vi "StartManageVIActivation.vi"(8 "error in (no error)":errorcluster, 11 "Menu in":refnum<class "VIActivation.lvclass">) -> (0 "error out":errorcluster, 3 "Menu out":refnum<class "VIActivation.lvclass">)   [LabVIEW 2021, in "VIActivation.lvlib" / "VIActivation.lvclass"]
uses:
  VIActivation.lvclass
  VIActivation.lvclass/VIActivation.ctl
  TR_ManageVIActivation.vi
  566083a2-3826-408d-bdf5-5786947dd1dc.vi
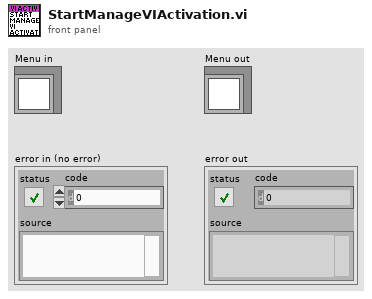
[diagram p1: front panel]
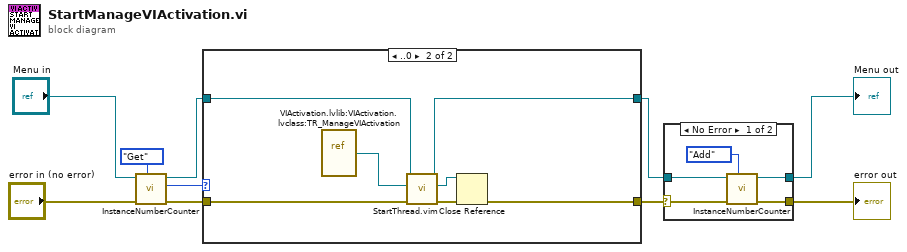
[diagram p0: block diagram]
diagram:
  n1 = call "InstanceNumberCounter.vi"("Action"=enum16{"Get", "Add", "Subtract"}."Get", "error in (no error)"="error in (no error)", "VI Activation in"="Menu in") -> ("error out"=w7:errorcluster, "InstanceNumber out"=w4:i32, "VI Activation out"=w2:refnum<class "VIActivation.lvclass">)  [unwired: 6 in]
  n2 = case shown="..0" w4 {
    tunnel: [w11 w14] -> w3
    tunnel: w7 -> [w11 w19]
    tunnel: w2 -> [w12 w17]
    tunnel: [w12 w16] -> w1
    frame Default {
    }
    frame ..0 {
      n3 = vi-ref "VIActivation.lvlib:VIActivation.lvclass:TR_ManageVIActivation.vi"() -> (w15:refnum<vi>)
      n4 = call "StartThread.vim"("error in (no error)"=w19, "VI Refnum in"=w15, "ByRefClass in"=w17) -> ("error out"=w18:errorcluster, "VI Refnum out"=w13:refnum<vi>, "ByRefClass out"=w16:refnum<class "VIActivation.lvclass">)  [unwired: 6 in]
      n5 = Close Reference(reference=w13, error in (no error)=w18) -> (error out=w14:errorcluster)
    }
  }
  n6 = case shown="No Error" w3 {
    selector: w3 -> [w20 w25]
    tunnel: [w24 w25] -> w10
    tunnel: [w23 w26] -> w9
    tunnel: w1 -> [w21 w26]
    frame No Error {
      n7 = call "InstanceNumberCounter.vi"("Action"=enum16{"Get", "Add", "Subtract"}."Add", "error in (no error)"=w20, "VI Activation in"=w21) -> ("error out"=w24:errorcluster, "VI Activation out"=w23:refnum<class "VIActivation.lvclass">)  [unwired: 6 in, 1 out]
    }
    frame Error {
    }
  }
  "Menu out" <- w9
  "error out" <- w10
